vi "Auto Release Frisbees (Mark Siekmeier's conflicted copy 2013-04-30).vi"() -> ()   [LabVIEW 2012]
uses:
  <vilib>/Rock Robotics/WPI/Solenoid/WPI_SolenoidValue.ctl
  <vilib>/Rock Robotics/WPI/Solenoid/WPI_SolenoidSetEnum.vi
  Robot Global Data.vi
panel:
  out "Loop Time 2":u32(graph)
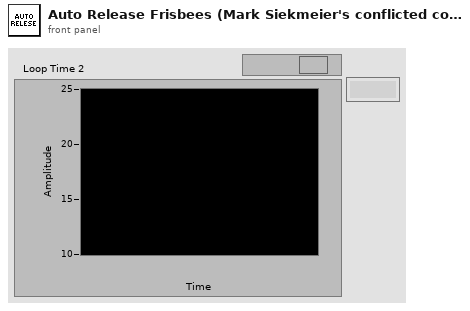
[diagram p1: front panel]
types:
  T1 = typedef "WPI_DigitalInputDevRef.ctl" = cluster{"DevStatus":errorcluster, "DIO Channel":T2, "Digital Module":T3}
  T2 = typedef "FPGA_DIOChannel.ctl" = enum8{"DIO 1", "DIO 2", "DIO 3", "DIO 4", "DIO 5", "DIO 6", "DIO 7", "DIO 8", "DIO 9", "DIO 10", "DIO 11", "DIO 12", "DIO 13", "DIO 14", "Invalid"}
  T3 = typedef "FPGA_TypedefDigitalModule.ctl" = enum16{"Digital Module 1", "Digital Module 2"}
  T4 = typedef "WPI_SolenoidDevRef.ctl" = cluster{"DevStatus":errorcluster, "Solenoid Module":T5, "Forward Solenoid Channel":T6, "Reverse Solenoid Channel":T6}
  T5 = typedef "FPGA_TypedefSolenoidModule.ctl" = enum16{"Solenoid Module 1", "Solenoid Module 2"}
  T6 = typedef "WPI_SolenoidChannel.ctl" = enum8{"Solenoid 1", "Solenoid 2", "Solenoid 3", "Solenoid 4", "Solenoid 5", "Solenoid 6", "Solenoid 7", "Solenoid 8", "Invalid"}
  T7 = typedef "WPI_SolenoidValue.ctl" = enum16{"Off", "On", "Forward", "Reverse"}
  T8 = enum16{"Spatula Down", "Not Fully Raised", "Up, None Released", "Up, One Released", "Up, Both Released", ""}
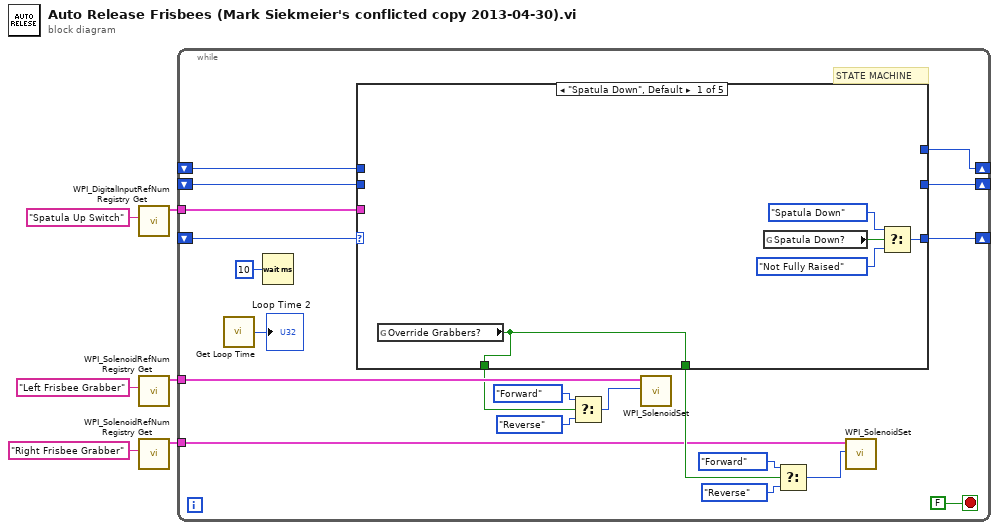
[diagram p0: block diagram]
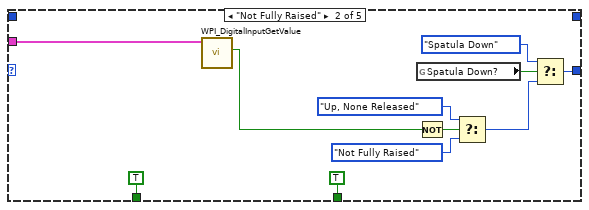
[diagram p2: hidden frame]
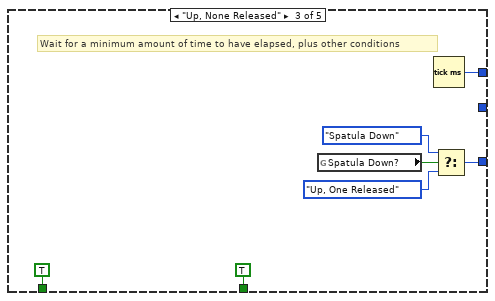
[diagram p3: hidden frame]
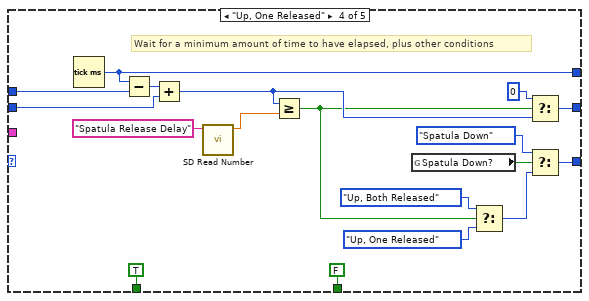
[diagram p4: hidden frame]
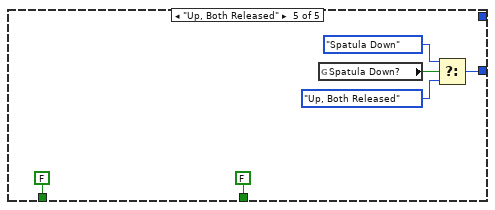
[diagram p5: hidden frame]
diagram:
  n1 = call <vilib>:"WPI_DigitalInputRefNum Registry Get.vi"("refnum name"="Spatula Up Switch") -> ("DigitalInputDevRef"=w1:T1)  [unwired: 9 in, 1 out]
  n2 = call <vilib>:"WPI_SolenoidRefNum Registry Get.vi"("refnum name"="Left Frisbee Grabber") -> ("SolenoidDevRef"=w5:T4)  [unwired: 9 in, 1 out]
  n3 = call <vilib>:"WPI_SolenoidRefNum Registry Get.vi"("refnum name"="Right Frisbee Grabber") -> ("SolenoidDevRef"=w3:T4)  [unwired: 9 in, 1 out]
  n4 = while {
    shift-right: [w18] -> _
    shift-left: _ -> [w19]
    shift-right: [w23] -> _
    shift-left: _ -> [w24]
    shift-right: [w21] -> _
    shift-left: _ -> [w22]
    tunnel: w5 -> [w17]
    tunnel: w3 -> [w8]
    tunnel: w1 -> [w7]
    stop <- FALSE stop-if-true
    # "STATE MACHINE"
    n5 = call "Get Loop Time.vi"() -> ("Loop Time"=→"Loop Time 2":u32)  [unwired: 1 in]
    n6 = Wait (ms)(milliseconds to wait=u32 10) -> ()  [unwired: 1 out]
    n7 = case shown="\"Spatula Down\", Default" w19 {
      tunnel: w24 -> [_ _ _ w54 _]
      tunnel: [_ _ w43 w50 _] -> w23
      tunnel: w22 -> [_ _ _ w53 _]
      tunnel: [_ _ _ w52 _] -> w21
      tunnel: [w27 TRUE ("Plunger Extended?") TRUE ("Plunger Extended?") FALSE ("Plunger Extended?") FALSE ("Plunger Extended?")] -> w9
      tunnel: [w29 w38 w46 w51 w70] -> w18
      tunnel: [w27 TRUE ("Plunger Extended?") TRUE ("Plunger Extended?") TRUE ("Plunger Extended?") FALSE ("Plunger Extended?")] -> w13
      tunnel: w7 -> [_ w37 _ _ _]
      frame "Spatula Down", Default {
        n8 = global read "Robot Global Data.vi" "Override Grabbers?"() -> (w27:bool)
        n9 = global read "Robot Global Data.vi" "Spatula Down?"() -> (w31:bool)
        n10 = Select(t=T8."Spatula Down" ("State"), s=w31, f=T8."Not Fully Raised") -> (s? t:f=w29:T8)
      }
      frame "Not Fully Raised" {
        n11 = call <vilib>:"WPI_DigitalInputGetValue.vi"("DigitalInputDevRef"=w37) -> ("Value"=w33:bool)  [unwired: 8 in, 2 out]
        n12 = global read "Robot Global Data.vi" "Spatula Down?"() -> (w40:bool)
        n13 = Not(x=w33) -> (.not. x?=w34:bool)
        n14 = Select(t=T8."Up, None Released" ("State"), s=w34, f=T8."Not Fully Raised" ("State")) -> (s? t:f=w35:T8)
        n15 = Select(t=T8."Spatula Down" ("State"), s=w40, f=w35) -> (s? t:f=w38:T8)
      }
      frame "Up, None Released" {
        # "Wait for a minimum amount of time to have elapsed, plus other conditions"
        n16 = global read "Robot Global Data.vi" "Spatula Down?"() -> (w49:bool)
        n17 = Tick Count (ms)() -> (millisecond timer value=w43:u32)
        n18 = Select(t=T8."Spatula Down" ("State"), s=w49, f=T8."Up, One Released" ("State")) -> (s? t:f=w46:T8)
      }
      frame "Up, One Released" {
        # "Wait for a minimum amount of time to have elapsed, plus other conditions"
        n19 = Tick Count (ms)() -> (millisecond timer value=w50:u32)
        n20 = Subtract(x=w50, y=w54) -> (x-y=w65:u32)
        n21 = Add(x=w65, y=w53) -> (x+y=w63:u32)
        n22 = call <vilib>:"SD Read Number.vi"("Name"="Spatula Release Delay") -> ("Numeric"=w61:dbl)  [unwired: 8 in, 2 out]
        n23 = Greater Or Equal?(x=w63, y=w61) -> (x >= y?=w57:bool)
        n24 = global read "Robot Global Data.vi" "Spatula Down?"() -> (w66:bool)
        n25 = Select(t=T8."Up, Both Released" ("State"), s=w57, f=T8."Up, One Released" ("State")) -> (s? t:f=w59:T8)
        n26 = Select(t=u32 0, s=w57, f=w63) -> (s? t:f=w52:u32)
        n27 = Select(t=T8."Spatula Down" ("State"), s=w66, f=w59) -> (s? t:f=w51:T8)
      }
      frame "Up, Both Released" {
        n28 = global read "Robot Global Data.vi" "Spatula Down?"() -> (w73:bool)
        n29 = Select(t=T8."Spatula Down" ("State"), s=w73, f=T8."Up, Both Released") -> (s? t:f=w70:T8)
      }
    }
    n30 = Select(t=WPI_SolenoidValue."Forward" ("Value"), s=w13, f=WPI_SolenoidValue."Reverse" ("Value")) -> (s? t:f=w15:T7)
    n31 = call-poly <vilib>:"WPI_SolenoidSet.vi"("Value"=w15, "SolenoidDevRef"=w17) -> ()  [unwired: 8 in, 2 out]
    n32 = Select(t=WPI_SolenoidValue."Forward" ("Value"), s=w9, f=WPI_SolenoidValue."Reverse" ("Value")) -> (s? t:f=w12:T7)
    n33 = call-poly <vilib>:"WPI_SolenoidSet.vi"("Value"=w12, "SolenoidDevRef"=w8) -> ()  [unwired: 8 in, 2 out]
  }
